vi "Linker Explorer UI.vi"() -> ()   [LabVIEW 2020, in "Linker Info.lvlib"]
uses:
  Linker Info.lvlib
  <vilib>/Utility/lvfile.llb/LVFileType.ctl
  <vilib>/Utility/lvfile.llb/NI_FileType.lvlib
panel:
  in  "Recursive":bool
  in  "File":path
  in  "Name Filter":string
  in  "Item Filter":string
  in  "Path Filter":string
  in  "Items":i32(listbox)
  in  "Tree":string(tree)
  out "Index":i32
  out "links":u32[](array[numeric])
  out "Linker Info":T2(array[cluster])
  out "Index Map":map{string, i32}(c390)
  out "Full Name":string
  out "viflags2":u32 format="%032b"
  out "viflags":u32 format="%032b"
  out "buttons":u16 format="%016b"
  out "wStyle":u16 format="%016b"
  out "iStyle":u16 format="%016b"
  out "iState":u32 format="%032b"
  out "Type":T1
  out "Path":path
  out "Status":string
  # "Selected Item"
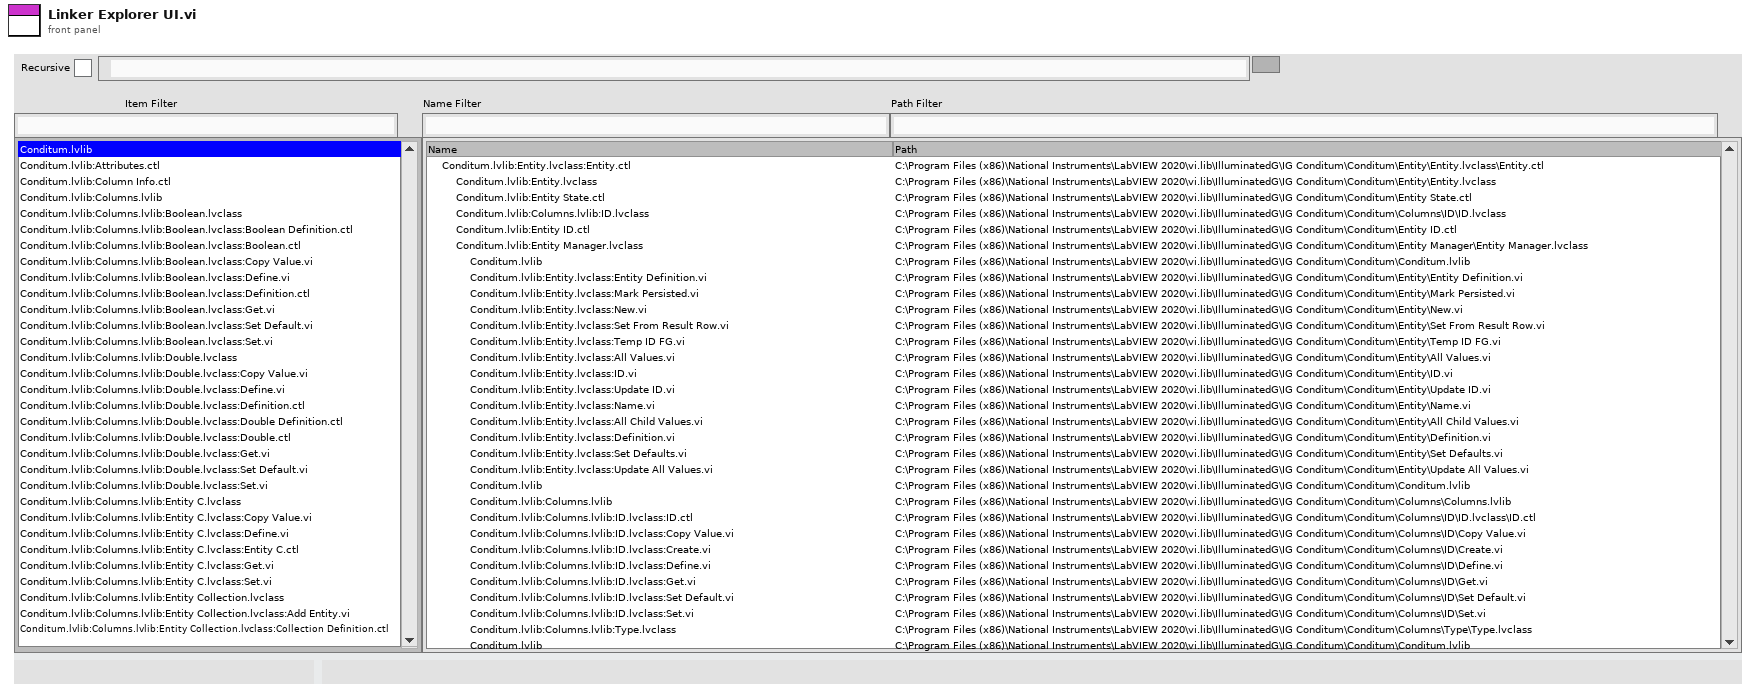
[diagram p1: front panel]
types:
  T1 = typedef "NI_FileType.lvlib/LVFileType.ctl" = enum32{"Invalid file", "Unknown type", "Instrument", "Control", "Polymorphic VI", "Project", "Library", "LVClass", "XControl", "XNode", "Shared library", ".NET assembly", "ActiveX interface", "CIN", "Run-time menu", "Palette menu", "Help file", "LLB", "XNode Edit Dependency", "Class Private Data Control", "Statechart", "MathScript .m file", "Ladder Diagram", "LVLibp", "XNode Build Dependency"}
  T2 = cluster{"path":path, "delimited name":string, "type":T1, "iState":u32, "iStyle":u16, "wStyle":u16, "buttons":u16, "viflags":u32, "viflags2":u32, "links":u32[]}[]
  T3 = cluster{"path":path, "delimited name":string, "type":T1, "iState":u32, "iStyle":u16, "wStyle":u16, "buttons":u16, "viflags":u32, "viflags2":u32, "links":u32[]}
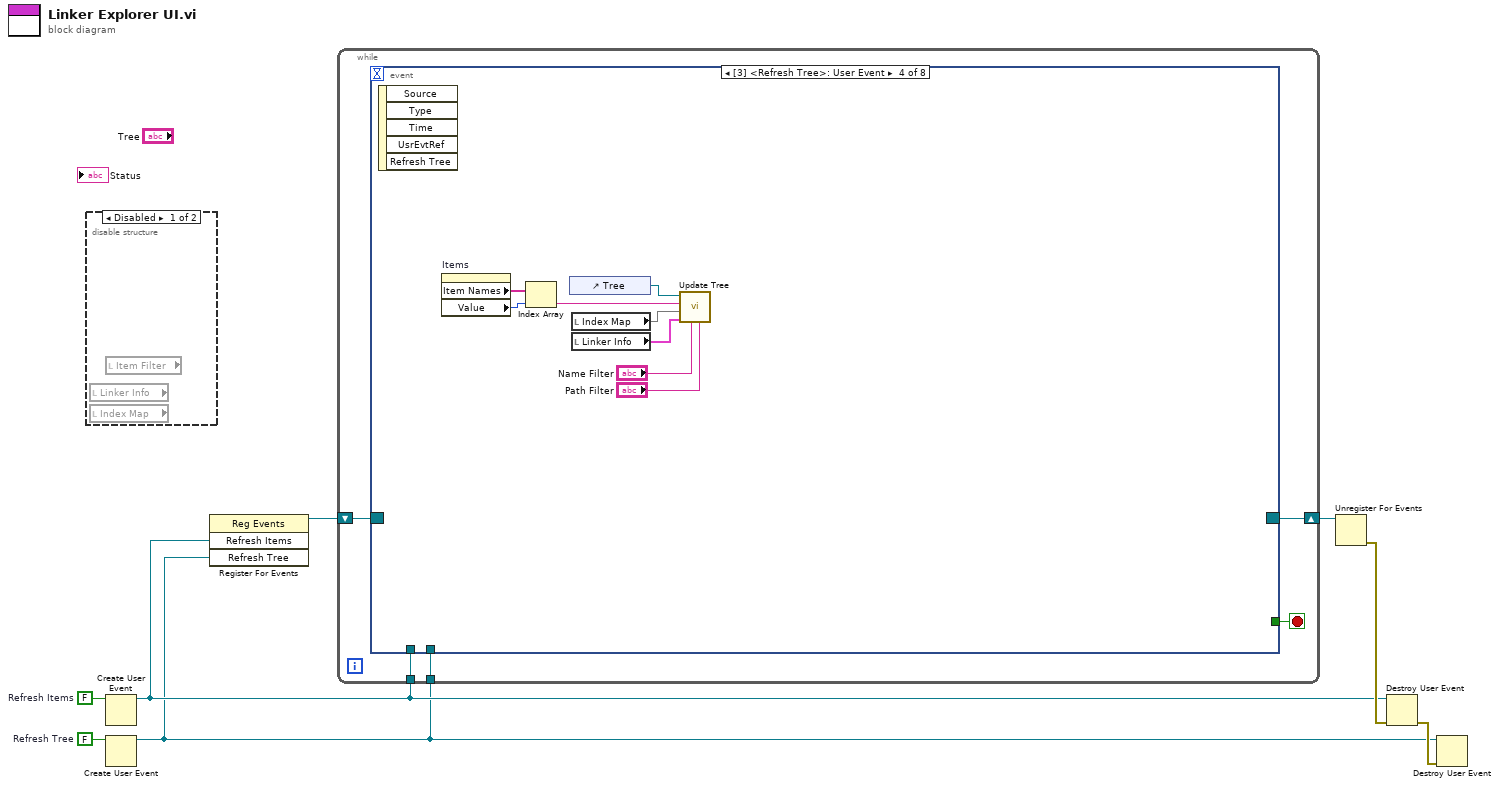
[diagram p0: block diagram]
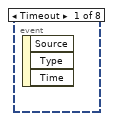
[diagram p3: hidden frame]
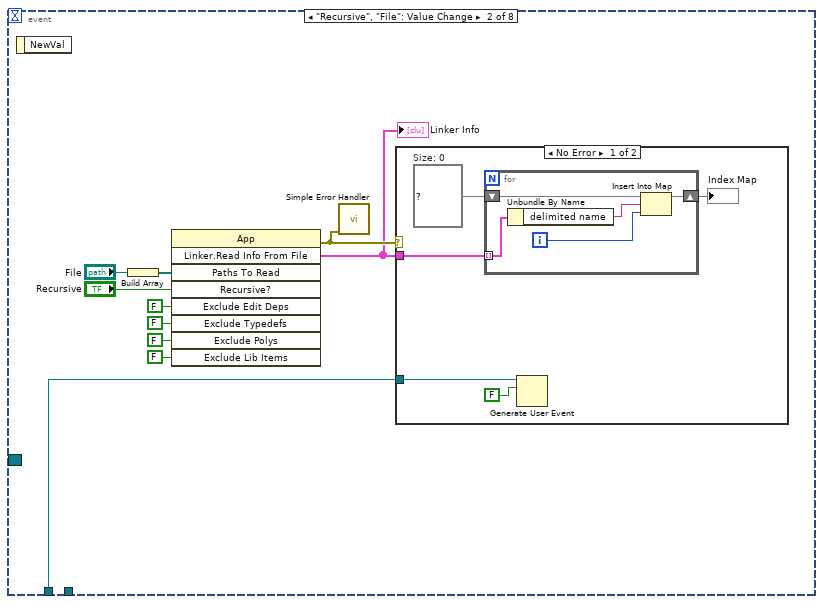
[diagram p4: hidden frame]
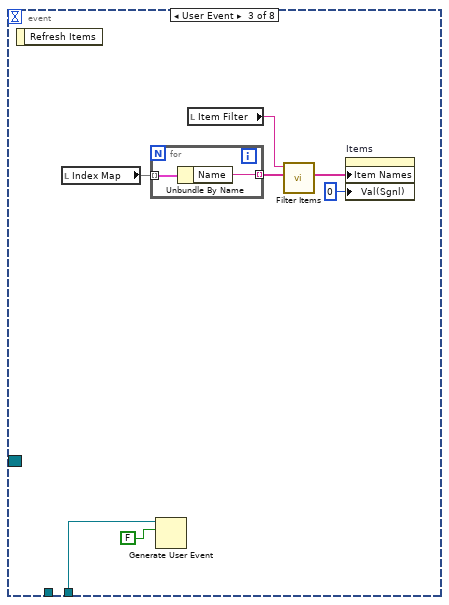
[diagram p6: hidden frame]
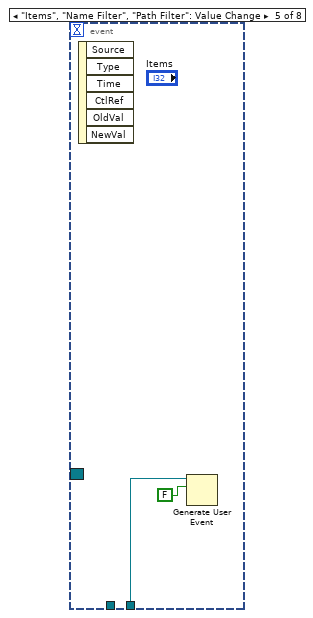
[diagram p7: hidden frame]
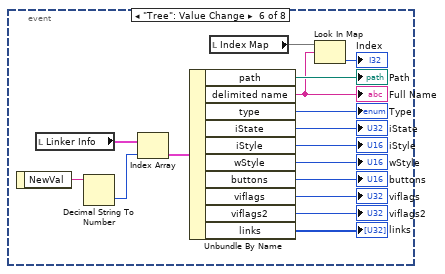
[diagram p8: hidden frame]
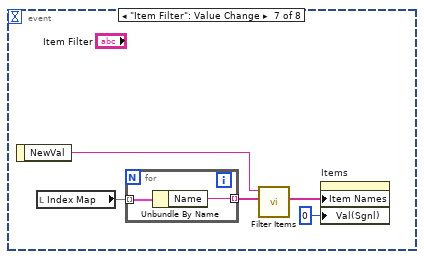
[diagram p9: hidden frame]
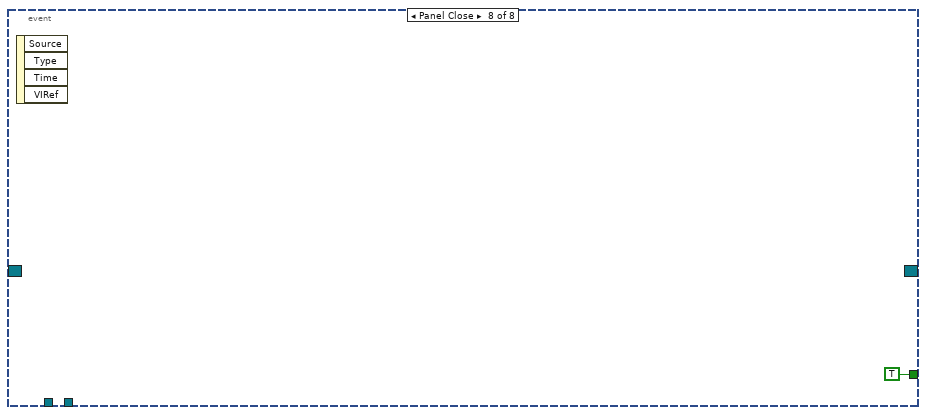
[diagram p10: hidden frame]
diagram:
  w3 = FALSE  # Refresh Tree
  w7 = FALSE  # Refresh Items
  n1 = disable-structure shown="Disabled" {
    frame Disabled {
      n2 = local read "Linker Info"() -> ()  [unwired: 1 out]
      n3 = local read "Index Map"() -> ()  [unwired: 1 out]
      n4 = local read "Item Filter"() -> ()  [unwired: 1 out]
    }
    frame Enabled {
    }
  }
  n5 = Create User Event(user event datatype=w7) -> (user event=w4:refnum<user-event>)  [unwired: 1 in, 1 out]
  n6 = Create User Event(user event datatype=w3) -> (user event=w1:refnum<user-event>)  [unwired: 1 in, 1 out]
  n7 = register-events(w4, w1) -> (reference out=w6:refnum<event-registration>)  [unwired: 2 in, 1 out]
  n8 = while {
    shift-right: [w10] -> w5
    shift-left: w6 -> [w12]
    tunnel: w4 -> [w11]
    tunnel: w1 -> [w9]
    stop <- w13 stop-if-true
    n9 = event shown="[3] <Refresh Tree>: User Event" {
      selector: w12 -> [_ _ _ _ _ _ _ _]
      dyn-events: [_ _ _ _ _ _ _ _] -> w10
      timeout: _ -> [_ _ _ _ _ _ _ _]
      tunnel: [_ _ _ _ _ _ _ TRUE] -> w13
      tunnel: w11 -> [_ w16 _ _ _ _ _ _]
      tunnel: w9 -> [_ _ w35 _ w52 _ _ _]
      event Timeout {
        n10 = event-data() -> ()  [unwired: 1 in, 3 out]
      }
      event "Recursive", "File": Value Change {
        n11 = event-data() -> ()  [unwired: 1 in, 1 out]
        n12 = Build Array("File") -> (w22:path[])
        n13 = invoke class="App" method="Linker.Read Info From File"("Paths To Read"=w22, "Recursive?"="Recursive", "Exclude Edit Deps"=FALSE ("Exclude Edit Time Dependencies"), "Exclude Typedefs"=FALSE, "Exclude Polys"=FALSE ("Exclude Poly VIs"), "Exclude Lib Items"=FALSE ("Exclude Unused Library Items")) -> (error out=w15:errorcluster, "Linker.Read Info From File"=w14:T2)  [unwired: 3 in, 7 out]
        "Linker Info" <- w14
        n14 = call <vilib>:"Simple Error Handler.vi"("error in (no error)"=w15) -> ()  [unwired: 4 in, 5 out]
        n15 = case shown="No Error" w15 {
          tunnel: w16 -> [w28 _]
          tunnel: w14 -> [w26 _]
          frame No Error {
            w25 = map{string, i32} {}  # Size: 0
            n16 = for {
              tunnel: w26 -> [w30] mode=indexing
              shift-right: [w32] -> w24
              shift-left: w25 -> [w33]
              i -> [w29]
              n17 = Unbundle By Name(w30) -> ("delimited name"=w31:string)
              n18 = Insert Into Map(map in=w33, key=w31, value=w29) -> (map out=w32:map{string, i32})  [unwired: 2 out]
            }
            "Index Map" <- w24
            n19 = Generate User Event(user event=w28, event data cluster=FALSE ("event data")) -> ()  [unwired: 2 in, 2 out]
          }
          frame Error {
          }
        }
      }
      event User Event {
        n20 = event-data() -> ()  [unwired: 1 in, 1 out]
        n21 = local read "Index Map"() -> (w40:map{string, i32})
        n22 = for {
          tunnel: w40 -> [w42] mode=indexing
          tunnel: [w41] -> w38 mode=indexing
          n23 = Unbundle By Name(w42) -> ("Name"=w41:string)
        }
        n24 = Generate User Event(user event=w35, event data cluster=FALSE ("event data")) -> ()  [unwired: 2 in, 2 out]
        n25 = local read "Item Filter"() -> (w36:string)
        n26 = call "Filter Items.vi"("Names"=w38, "Filter"=w36) -> ("Filtered Names"=w37:string[])  [unwired: 9 in]
        n27 = property on="Items" class="LstBox (strict)"("Item Names"=w37, "Val(Sgnl)"=0 ("Value (Signaling)")) -> ()  [unwired: 2 in, 2 out]
      }
      event User Event {
        n28 = event-data() -> ()  [unwired: 1 in, 5 out]
        n29 = property on="Items" class="LstBox (strict)"() -> ("Item Names"=w50:string[], "Value"=w49:i32)  [unwired: 2 in, 2 out]
        n30 = Index Array(array=w50, index=w49) -> (element=w47:string)
        n31 = control-ref of="Tree"() -> (w48:refnum<vi>)
        n32 = local read "Index Map"() -> (w46:map{string, i32})
        n33 = local read "Linker Info"() -> (w45:T2)
        n34 = call "Update Tree.vi"("Path Filter"="Path Filter", "Name Filter"="Name Filter", "Linker Info"=w45, "Index Map"=w46, "Item"=w47, "Tree In"=w48) -> ()  [unwired: 6 in]
      }
      event "Items", "Name Filter", "Path Filter": Value Change {
        n35 = event-data() -> ()  [unwired: 1 in, 6 out]
        n36 = Generate User Event(user event=w52, event data cluster=FALSE ("event data")) -> ()  [unwired: 2 in, 2 out]
      }
      event "Tree": Value Change {
        n37 = event-data() -> ("NewVal"=w68:string)  [unwired: 1 in]
        n38 = local read "Linker Info"() -> (w67:T2)
        n39 = Decimal String To Number(string=w68) -> (number=w66:i32)  [unwired: 2 in, 1 out]
        n40 = Index Array(array=w67, index=w66) -> (element=w65:T3)
        n41 = Unbundle By Name(w65) -> ("path"=→"Path":path, "delimited name"=w54:string, "type"=→"Type":T1, "iState"=→"iState":u32, "iStyle"=→"iStyle":u16, "wStyle"=→"wStyle":u16, "buttons"=→"buttons":u16, "viflags"=→"viflags":u32, "viflags2"=→"viflags2":u32, "links"=→"links":u32[])
        "Full Name" <- w54
        n42 = local read "Index Map"() -> (w55:map{string, i32})
        n43 = Look In Map(map=w55, key=w54) -> (value=→"Index":i32)  [unwired: 1 in, 1 out]
      }
      event "Item Filter": Value Change {
        n44 = event-data() -> ("NewVal"=w69:string)  [unwired: 1 in]
        n45 = local read "Index Map"() -> (w73:map{string, i32})
        n46 = for {
          tunnel: w73 -> [w75] mode=indexing
          tunnel: [w74] -> w72 mode=indexing
          n47 = Unbundle By Name(w75) -> ("Name"=w74:string)
        }
        n48 = call "Filter Items.vi"("Names"=w72, "Filter"=w69) -> ("Filtered Names"=w71:string[])  [unwired: 9 in]
        n49 = property on="Items" class="LstBox (strict)"("Item Names"=w71, "Val(Sgnl)"=0 ("Value (Signaling)")) -> ()  [unwired: 2 in, 2 out]
      }
      event Panel Close {
        n50 = event-data() -> ()  [unwired: 1 in, 4 out]
      }
    }
  }
  n51 = Unregister For Events(event registration refnum=w5) -> (error out=w8:errorcluster)  [unwired: 1 in]
  n52 = Destroy User Event(user event=w4, error in=w8) -> (error out=w2:errorcluster)
  n53 = Destroy User Event(user event=w1, error in=w2) -> ()  [unwired: 1 out]
